vi "Move Impl.vi"(6 "Mode":enum16{"Relative", "Absolute"}(ring), 8 "error in (no error)":errorcluster, 9 "Value (um)":dbl format="%#_13g", 10 "Axis":T1=enum."Y", 11 "Newport ESP301 Stage in":refnum<class "Newport ESP301 Stage.lvclass">) -> (0 "error out":errorcluster, 3 "Newport ESP301 Stage out":refnum<class "Newport ESP301 Stage.lvclass">)   [LabVIEW 2023, in "Newport ESP301 Stage.lvlib" / "Newport ESP301 Stage.lvclass"]
uses:
  Newport ESP301 Stage.lvclass
  Stage Controller/Stage Axis.ctl
  Newport ESP301 Stage.lvclass/Newport ESP301 Stage.ctl
  Stage Controller/Stage Controller.lvclass
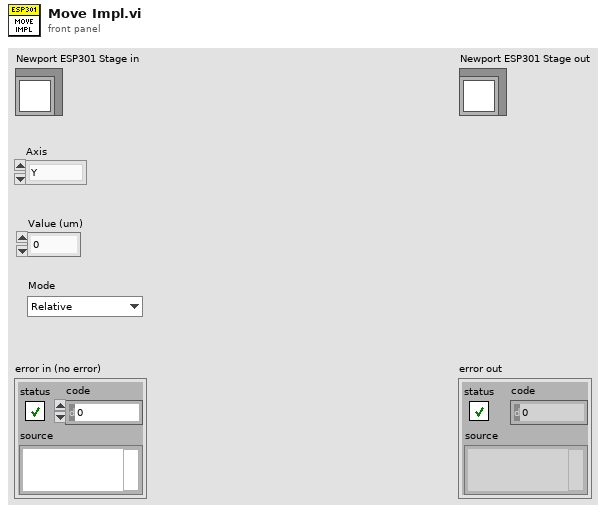
[diagram p1: front panel]
types:
  T1 = typedef "Stage Controller.lvlib/Stage Controller.lvclass/Stage Axis.ctl" = enum16{"unspecified", "X", "Y", "Z"}
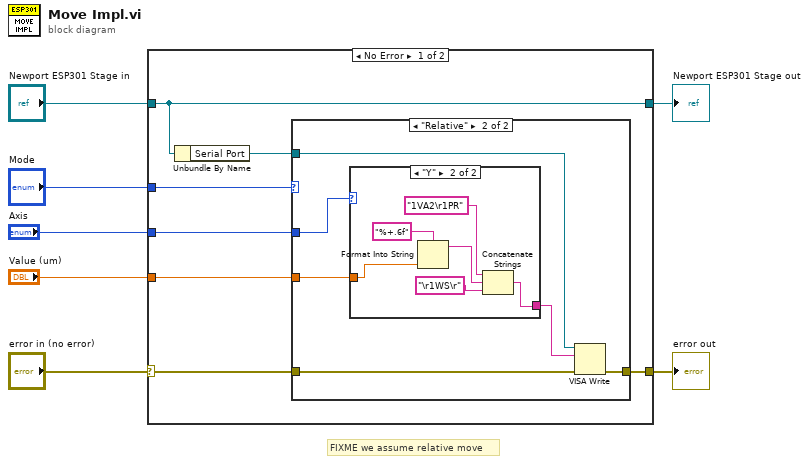
[diagram p0: block diagram]
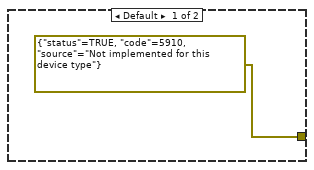
[diagram p2: hidden frame]
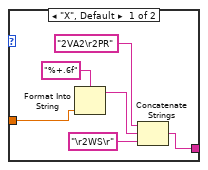
[diagram p3: hidden frame]
diagram:
  # "FIXME we assume relative move"
  n1 = case shown="No Error" "error in (no error)" {
    selector: "error in (no error)" -> [w9 w34]
    tunnel: "Newport ESP301 Stage in" -> [w14 w35]
    tunnel: [w14 w35] -> w5
    tunnel: [w8 w34] -> w4
    tunnel: "Mode" -> [w11 _]
    tunnel: "Axis" -> [w13 _]
    tunnel: "Value (um)" -> [w12 _]
    frame No Error {
      n2 = Unbundle By Name(w14) -> ("Serial Port"=w10:refnum<visa-resource-name>)
      n3 = case shown="\"Relative\"" w11 {
        tunnel: w13 -> [_ w21]
        tunnel: w12 -> [_ w20]
        tunnel: w10 -> [_ w17]
        tunnel: w9 -> [_ w19]
        tunnel: [errorcluster {"status"=TRUE, "code"=5910, "source"="Not implemented for this device type"} ("error IO") w18] -> w8
        frame Default {
        }
        frame "Relative" {
          n4 = case shown="\"Y\"" w21 {
            tunnel: w20 -> [w22 w29]
            tunnel: [w25 w28] -> w16
            frame "X", Default {
              n5 = Format Into String(format string="%+.6f", w22) -> (resulting string=w24:string)  [unwired: 2 in, 1 out]
              n6 = Concatenate Strings("2VA2\r2PR" ("write buffer"), w24, "\r2WS\r" ("write buffer")) -> (w25:string)
            }
            frame "Y" {
              n7 = Format Into String(format string="%+.6f", w29) -> (resulting string=w33:string)  [unwired: 2 in, 1 out]
              n8 = Concatenate Strings("1VA2\r1PR" ("write buffer"), w33, "\r1WS\r" ("write buffer")) -> (w28:string)
            }
          }
          n9 = VISA Write(VISA resource name=w17, write buffer=w16, error in (no error)=w19) -> (error out=w18:errorcluster)  [unwired: 2 out]
        }
      }
    }
    frame Error {
    }
  }
  "error out" <- w4
  "Newport ESP301 Stage out" <- w5
